vi "McPherson Setup.vi"(2 "Setup(F)Close(T)":bool, 5 "VISA resource name":refnum<visa-resource-name>) -> (0 "error out":errorcluster, 1 "Setpoint":dbl format="%.2f")   [LabVIEW 2024]
uses:
  Serial Instruments/Serial Support VISA.llb/Serial Actions.ctl
  Globals and TypeDefs/Global Varibal Control.vi
panel:
  out "X-Axis Unit String":string
  out "UnitFormatString":string="nm"
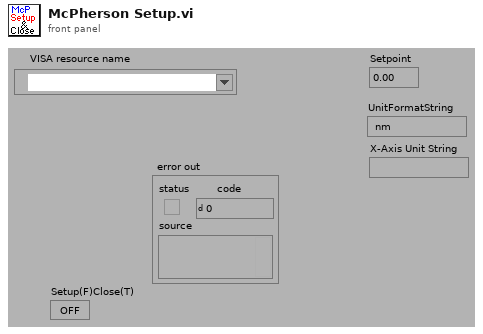
[diagram p1: front panel]
types:
  T1 = typedef "Serial Actions.ctl" = enum16{"Init", "Break", "Clear Buffer", "Write", "Read", "N Bytes", "Lock", "Unlock", "Close"}
  T2 = cluster{"StepperPosition":i32, "MovingStatus":i32, "V":i32, "K":i32, "I":i32}
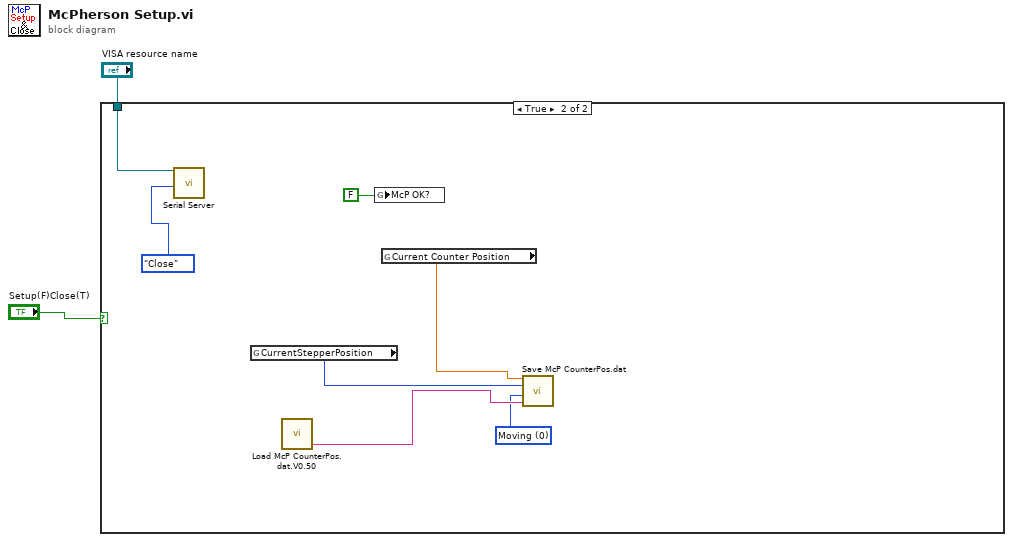
[diagram p0: block diagram]
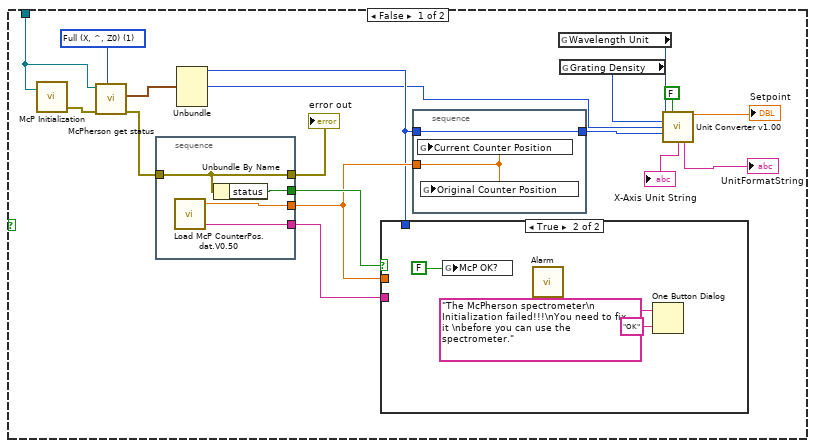
[diagram p2: hidden frame]
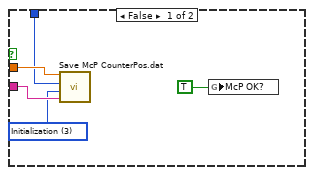
[diagram p3: hidden frame]
diagram:
  n1 = case shown="True" "Setup(F)Close(T)" {
    tunnel: "VISA resource name" -> [w3 w35]
    frame False {
      w4 = u16 1 items=["Grab Globals", "Full (X, ^, Z0)", "Moving(^ and Z0)", "Position(Z0)"] ("Status")
      n2 = call "McP Initialization.vi"("VISA resource name"=w3) -> ("error out"=w20:errorcluster)  [unwired: 1 in, 2 out]
      n3 = call "McPherson get status.vi"("Status"=w4, "error in (no error)"=w20, "VISA Resource Name"=w3) -> ("error out"=w19:errorcluster, "StatusParameter"=w7:T2)  [unwired: 2 in, 2 out]
      n4 = stacked-sequence {
        tunnel: [w32] -> w17
        tunnel: w19 -> [w32]
        tunnel: [w34] -> w15
        tunnel: [w33] -> w18
        tunnel: [w31] -> w16
        frame #0 {
          n5 = call "Load McP CounterPos.dat.V0.50.vi"() -> ("Counter Position"=w34:dbl, "Last Calibration Date"=w33:string)  [unwired: 1 in, 1 out]
          n6 = Unbundle By Name(w32) -> ("status"=w31:bool)
        }
      }
      "error out" <- w17
      n7 = Unbundle(w7) -> ("StepperPosition"=w6:i32, "V"=w5:i32)  [unwired: 3 out]
      n8 = case shown="True" w16 {
        tunnel: w18 -> [w27 _]
        tunnel: w15 -> [w26 _]
        tunnel: w6 -> [w25 _]
        frame False {
          w24 = u16 3 items=["Moving", "Calibration", "Key in", "Initialization"] ("Set Method")
          n9 = call "Save McP CounterPos.dat.vi"("Last Calibration Date"=w27, "Set Method"=w24, "McP Stepper Position"=w25, "McP Counter Position"=w26) -> ()  [unwired: 2 in, 1 out]
          n10 = global write "Global Varibal Control.vi" "McP OK?"(TRUE ("McP OK?")) -> ()
        }
        frame True {
          n11 = global write "Global Varibal Control.vi" "McP OK?"(FALSE ("McP OK?")) -> ()
          n12 = call "Alarm.vi"() -> ()  [unwired: 4 in]
          n13 = One Button Dialog(message="The McPherson spectrometer\n Initialization failed!!!\nYou need to fix it \nbefore you can use the spectrometer.", button name ("OK")="OK") -> ()  [unwired: 1 out]
        }
      }
      n14 = stacked-sequence {
        tunnel: w15 -> [w21]
        tunnel: [w22] -> w9
        tunnel: w6 -> [w22]
        frame #0 {
          n15 = global write "Global Varibal Control.vi" "Current Counter Position"(w21) -> ()
          n16 = global write "Global Varibal Control.vi" "Original Counter Position"(w21) -> ()
        }
      }
      n17 = global read "Global Varibal Control.vi" "Wavelength Unit"() -> (w14:u8)
      n18 = global read "Global Varibal Control.vi" "Grating Density"() -> (w13:u8)
      n19 = call "Unit Converter v1.00.vi"("Wavelength Unit"=w14, "x to W (F) or W to x (T)"=FALSE, "Grating Density"=w13, "Velocity (Steps/s)"=w5, "Stepper Position Input"=w9) -> ("Wavelength Output"=→"Setpoint":dbl, "X-Axis Unit String"=→"X-Axis Unit String":string, "UnitFormatString"=→"UnitFormatString":string)  [unwired: 3 in, 5 out]
    }
    frame True {
      w40 = u16 0 items=["Moving", "Calibration", "Key in", "Initialization"] ("Set Method")
      n20 = call "Serial Server.vi"("VISA Resource Name"=w35, "Action"=Serial_Actions."Close") -> ()  [unwired: 9 in, 5 out]
      n21 = global read "Global Varibal Control.vi" "CurrentStepperPosition"() -> (w37:i32)
      n22 = call "Load McP CounterPos.dat.V0.50.vi"() -> ("Last Calibration Date"=w41:string)  [unwired: 1 in, 2 out]
      n23 = global write "Global Varibal Control.vi" "McP OK?"(FALSE ("McP OK?")) -> ()
      n24 = global read "Global Varibal Control.vi" "Current Counter Position"() -> (w38:dbl)
      n25 = call "Save McP CounterPos.dat.vi"("Last Calibration Date"=w41, "Set Method"=w40, "McP Stepper Position"=w37, "McP Counter Position"=w38) -> ()  [unwired: 2 in, 1 out]
    }
  }
